vi "Add Timing Section.vi"(8 "error in":errorcluster, 11 "custom device ref":T1 format="%.0x") -> (0 "error out":errorcluster, 2 "timing":T1 format="%.0x", 3 "custom device ref out":T1 format="%.0x")   [LabVIEW 2020, in "AIM ARINC 429 Scripting.lvlib"]
uses:
  <vilib>/NI VeriStand/Custom Device API/Custom Device Item Ref.ctl
  Constants.vi
  AIM ARINC 429 Scripting.lvlib
  <vilib>/NI VeriStand/Custom Device API/Custom Device API.lvlib
  <vilib>/NI VeriStand/Custom Device API/Custom Device Channel Type.ctl
  <vilib>/NI VeriStand/Custom Device API/Custom Device Channel.ctl
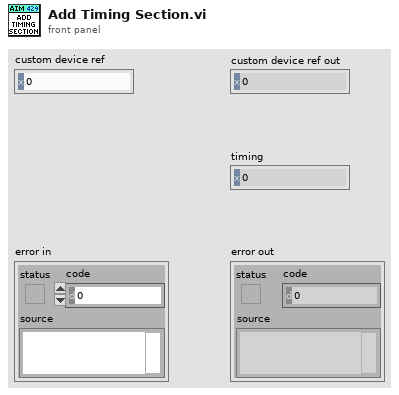
[diagram p1: front panel]
types:
  T1 = typedef "Custom Device API.lvlib/Custom Device Item Ref.ctl" = u64
  T2 = typedef "Custom Device API.lvlib/Custom Device Channel.ctl" = cluster{"Type":T3, "Units":string, "Default Value":dbl, "Faultable":bool, "Scalable":bool}
  T3 = typedef "Custom Device API.lvlib/Custom Device Channel Type.ctl" = enum16{"Input", "Output"}
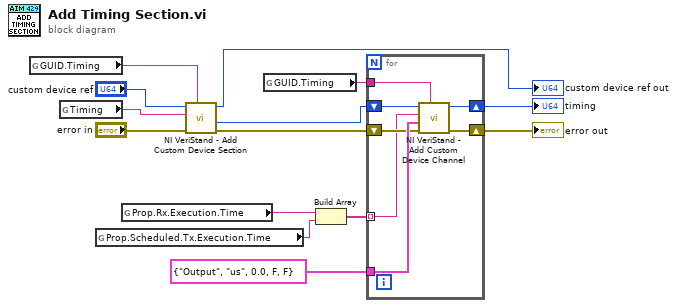
[diagram p0: block diagram]
diagram:
  n1 = global read "Constants.vi" "GUID.Timing"() -> (w12:string)
  n2 = global read "Constants.vi" "Timing"() -> (w11:string)
  n3 = global read "Constants.vi" "Prop.Scheduled.Tx.Execution.Time"() -> (w1:string)
  n4 = global read "Constants.vi" "Prop.Rx.Execution.Time"() -> (w2:string)
  n5 = call <vilib>:"NI VeriStand - Add Custom Device Section.vi"("GUID (Default Section)"=w12, "error in (no error)"="error in", "Section Name"=w11, "Parent Ref in"="custom device ref") -> ("error out"=w8:errorcluster, "Section Ptr"=w6:T1, "Parent Ref out"=→"custom device ref out":T1)  [unwired: 4 in, 1 out]
  n6 = global read "Constants.vi" "GUID.Timing"() -> (w3:string)
  n7 = Build Array(w2, w1) -> (w9:string[])
  n8 = for {
    tunnel: w3 -> [w20]
    tunnel: T2 {"Type"=enum."Output", "Units"="us", "Default Value"=0.0, "Faultable"=FALSE, "Scalable"=FALSE} ("Channel") -> [w19]
    shift-right: [w16] -> w4
    shift-left: w6 -> [w21]
    shift-right: [w17] -> w7
    shift-left: w8 -> [w18]
    tunnel: w9 -> [w15] mode=indexing
    n9 = call <vilib>:"NI VeriStand - Add Custom Device Channel.vi"("GUID (Default Channel)"=w20, "error in (no error)"=w18, "Channel"=w19, "Channel Name"=w15, "Parent Ref in"=w21) -> ("error out"=w17:errorcluster, "Parent Ref out"=w16:T1)  [unwired: 3 in, 2 out]
  }
  "error out" <- w7
  "timing" <- w4
